vi "AT Delete Buffer A.vi"(8 "error in (no error)":errorcluster, 10 "Buffer":u64, 11 "Handle":u32) -> (0 "error out":errorcluster, 3 "Status":i32)   [LabVIEW 2009]
doc: "DeleteBuffer\n\nOutput:\n I32 Status\n\nInput:\n I32 Handle\n U8 buffer\n\nDeletes the buffer and frees the allocated memory."
uses:
  atcoreA.dll
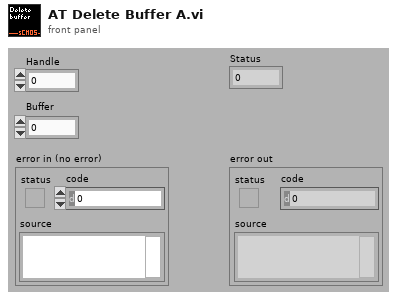
[diagram p1: front panel]
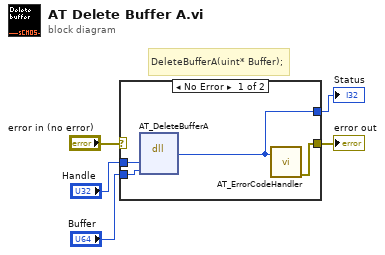
[diagram p0: block diagram]
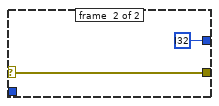
[diagram p2: hidden frame]
diagram:
  # "DeleteBufferA(uint* Buffer);"
  n1 = case shown="No Error" "error in (no error)" {
    selector: "error in (no error)" -> [_ w11]
    tunnel: "Buffer" -> [w9 _]
    tunnel: [w6 i32 ?] -> w3
    tunnel: [w7 w11] -> w2
    tunnel: "Handle" -> [w8 _]
    frame #0 {
      n2 = dll-call lib="atcoreA.dll" fn="AT_DeleteBufferA"("Handle"=w8, "Buffer"=w9) -> ("Status"=w6:i32)  [unwired: 5 in, 2 out]
      n3 = call "AT_ErrorCodeHandler.vi"("Error"=w6) -> ("error out"=w7:errorcluster)  [unwired: 6 in]
    }
    frame #1 {
    }
  }
  "Status" <- w3
  "error out" <- w2
